vi "Array of VData to VCluster_openG.vi"(8 "error in (no error)":errorcluster, 11 "Array":variant[](array[variant])) -> (0 "error out":errorcluster, 3 "VCluster":variant)   [LabVIEW 2018, in "Tag Engine.lvlib"]
doc: "_SubVI_"
uses:
  Tag Engine.lvlib
panel:
  # "Slightly modified version of Array of VData to VCluster from OpenG"
  # "Array of VData to VCluster.vi\n\nReturns the elements of an array as elements of a variant cluster.\n\nPlease visit http://www.OpenG.org to learn about the\nOpen Source LabVIEW software movement.\n\nNOTICE -- YOU MUST LEAVE THIS NOTICE IN PLACE.  PER THE TERMS OF THE LICENSE BELOW, YOU MAY SUBLICENSE THIS SOFTWARE \nIN ANY WAY THAT DOES NOT CONFLICT WITH THIS LICENSE.\n\n### BSD License (http://www.opensource.org/licenses/bsd-license.php) Begin ###\n \nCopyright (c) 2002, Jean-Pierre Drolet <drolet_jp@hotmail.com>\nCopyright (c) 2002-2006, Jim Kring <jim@jimkring.com>\n\nAll rights reserved.\n\nRedistribution and use in source and binary forms, with or without modification, are permitted provided that the following conditions are met:\n\n    * Redistributions of source code must retain the above copyright notice, this list of conditions and the following disclaimer.\n    * Redistributions in binary form must reproduce the above copyright notice, this list of conditions and the following disclaimer in the \n       documentation and/or other materials provided with the distribution.\n    * Neither the name of SciWare, James Kring, Inc., nor the names of its contributors may be used to endorse or promote products derived \n       from this software without specific prior written permission.\n\nTHIS SOFTWARE IS PROVIDED BY THE COPYRIGHT HOLDERS AND CONTRIBUTORS \"AS IS\" AND ANY EXPRESS OR IMPLIED WARRANTIES, \nINCLUDING, BUT NOT LIMITED TO, THE IMPLIED WARRANTIES OF MERCHANTABILITY AND FITNESS FOR A PARTICULAR PURPOSE ARE \nDISCLAIMED. IN NO EVENT SHALL THE COPYRIGHT OWNER OR CONTRIBUTORS BE LIABLE FOR ANY DIRECT, INDIRECT, INCIDENTAL,\n SPECIAL, EXEMPLARY, OR CONSEQUENTIAL DAMAGES (INCLUDING, BUT NOT LIMITED TO, PROCUREMENT OF SUBSTITUTE GOODS OR \nSERVICES; LOSS OF USE, DATA, OR PROFITS; OR BUSINESS INTERRUPTION) HOWEVER CAUSED AND ON ANY THEORY OF LIABILITY, \nWHETHER IN CONTRACT, STRICT LIABILITY, OR TORT (INCLUDING NEGLIGENCE OR OTHERWISE) ARISING IN ANY WAY OUT OF THE USE \nOF THIS SOFTWARE, EVEN IF ADVISED OF THE POSSIBILITY OF SUCH DAMAGE.\n\n### BSD License End ###"
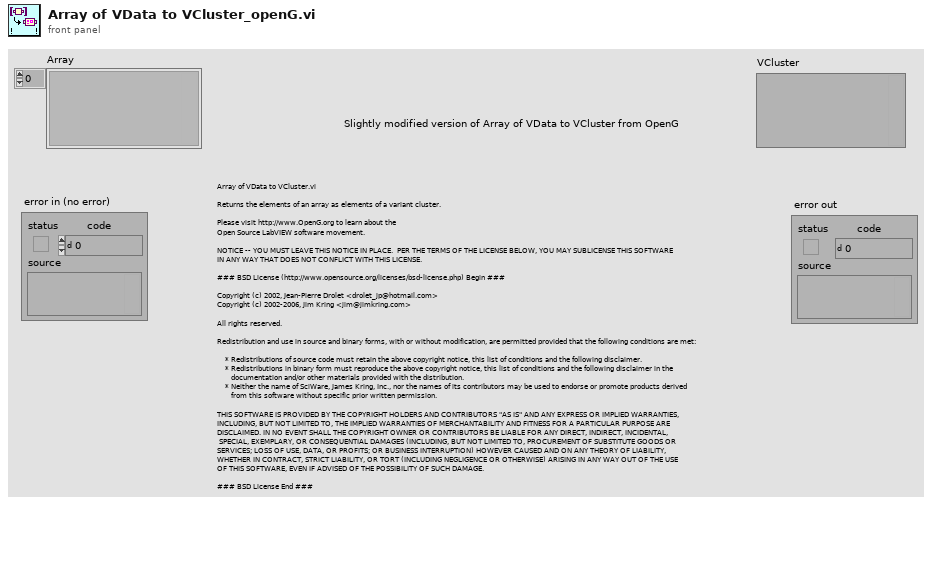
[diagram p1: front panel]
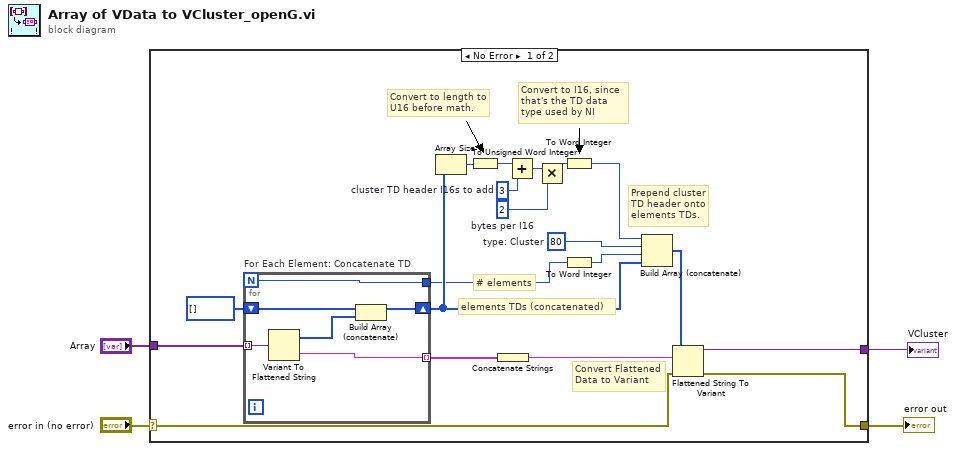
[diagram p0: block diagram]
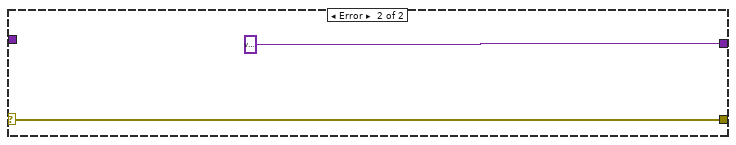
[diagram p2: hidden frame]
diagram:
  n1 = case shown="No Error" "error in (no error)" {
    selector: "error in (no error)" -> [w6 w31]
    tunnel: [w13 w31] -> w4
    tunnel: [w14 variant ("Variant")] -> w2
    tunnel: "Array" -> [w15 _]
    frame No Error {
      w5 = i16 80  # type: Cluster
      w9 = u16 2  # bytes per I16
      w11 = u16 3  # cluster TD header I16s to add
      # "Convert Flattened Data to Variant"
      # "elements TDs (concatenated)"
      # "Convert to length to U16 before math."
      # "Convert to I16, since that's the TD data type used by NI"
      # "Prepend cluster TD header onto elements TDs."
      # "# elements"
      n2 = for "For Each Element: Concatenate TD" {
        N -> [w27]
        tunnel: w15 -> [w26] mode=indexing
        tunnel: [w24] -> w23 mode=indexing
        shift-right: [w29] -> w17
        shift-left: i16[] [] -> [w28]
        tunnel: [w27] -> w12
        n3 = Variant To Flattened String(Variant=w26) -> (data string=w24:string, 1:w25:i16[])
        n4 = Build Array (concatenate)(w28, w25) -> (w29:i16[])
      }
      n5 = Array Size(array=w17) -> (size(s)=w19:i32)
      n6 = To Unsigned Word Integer(number=w19) -> (unsigned 16bit integer=w8:u16)
      n7 = Concatenate Strings(w23) -> (w21:string)
      n8 = Add(x=w8, y=w11) -> (x+y=w10:u16)
      n9 = Multiply(x=w10, y=w9) -> (x*y=w7:u16)
      n10 = To Word Integer(number=w7) -> (16bit integer=w18:i16)
      n11 = To Word Integer(number=w12) -> (16bit integer=w16:i16)
      n12 = Build Array (concatenate)(w18, w5, w16, w17) -> (w20:i16[])
      n13 = Flattened String To Variant(4:w6, 6:w21, 7:w20) -> (0:w13:errorcluster, 3:w14:variant)
    }
    frame Error {
    }
  }
  "error out" <- w4
  "VCluster" <- w2
